vi "Washing_Machine.vi"() -> ()   [LabVIEW 2021]
uses:
  Controls/Queue_Operation_Select.ctl
  Controls/State_and_Data.ctl
  Controls/Timer_Operation_Select.ctl
  Controls/INI_Operation_Select.ctl
  <vilib>/Utility/file.llb/Read Delimited Spreadsheet (string).vi
  8107810c-38f5-4bb1-a673-e4c5686a5b40.vi
  Controls/Wash_Type.ctl
panel:
  out "Elapsed_Time":dbl=1044.1757565 caption="Elapsed Time"
  out "Wash_Complete?":bool caption="Wash Complete?"
  out "Dry_Water":bool
  out "Short_Wash/Soak":bool
  out "Cool_Down":bool
  out "Regular":bool
  out "Machine_Underweight":bool
  out "Machine_Overweight":bool
  out "Machine_Load":dbl(slide) caption="Machine Load" scale=0.0..15.0
  in  "Unload":bool
  in  "Stop_Wash":bool
  in  "Start_Wash":bool
  in  "Wash_Type":T1 caption="Wash Type" scale=0.0..2.0
  in  "Add_Clothes":bool
  in  "Clothes [Kg]":dbl min=0.0 max=15.0
  out "Error_Out":errorcluster
  in  "Error_In":errorcluster
  # "Load Status"
  # "Sequence"
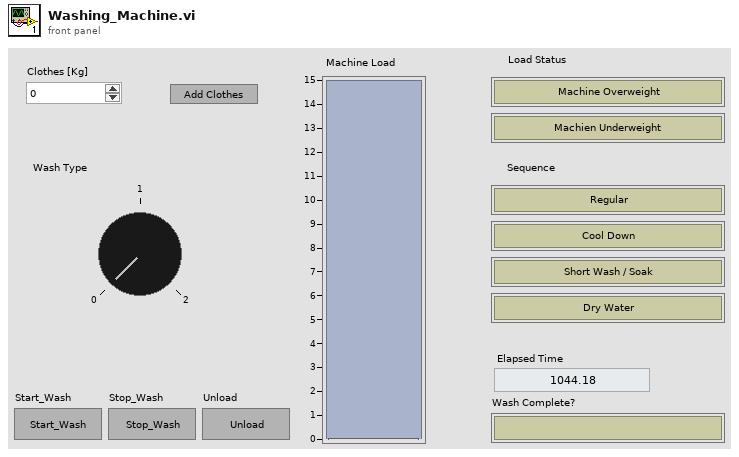
[diagram p1: front panel]
types:
  T1 = typedef "Wash_Type.ctl" = i32
  T2 = typedef "Timer_Operation_Select.ctl" = enum16{"Start_Timer", "Time_Out?", "Pause_Timer", "Stop_Timer"}
  T3 = typedef "State_and_Data.ctl" = cluster{"State":string, "Data":variant}
  T4 = typedef "Queue_Operation_Select.ctl" = enum16{"Obtain_Queue", "Enqueue", "Enqueue_First", "Enqueue_N", "Lossy_Enqueue", "Preview", "Queue_Status", "Dequeue", "Flush", "Release_Queue"}
  T5 = typedef "INI_Operation_Select.ctl" = enum16{"Initialize", "Read", "Write"}
  T6 = cluster{"Machine_Load":dbl, "Machine_Overweight":bool, "Machine_Underweight":bool, "Sequence":bool[], "Washing_Complete?":bool, "Disabled":enum8{"Enabled", "Disabled", "Disabled and Grayed Out"}, "Wash_Type":string, "Washing_Process":string[], "Process_Time":dbl[], "CSV_File_Path":path, "Current_Washing_Stage":i32, "Start?":bool, "Total_Washing_Stage":i32, "Washing_Process_F":bool[], "Machine_Load_Added":bool}
  T7 = enum8{"Enabled", "Disabled", "Disabled and Grayed Out"}
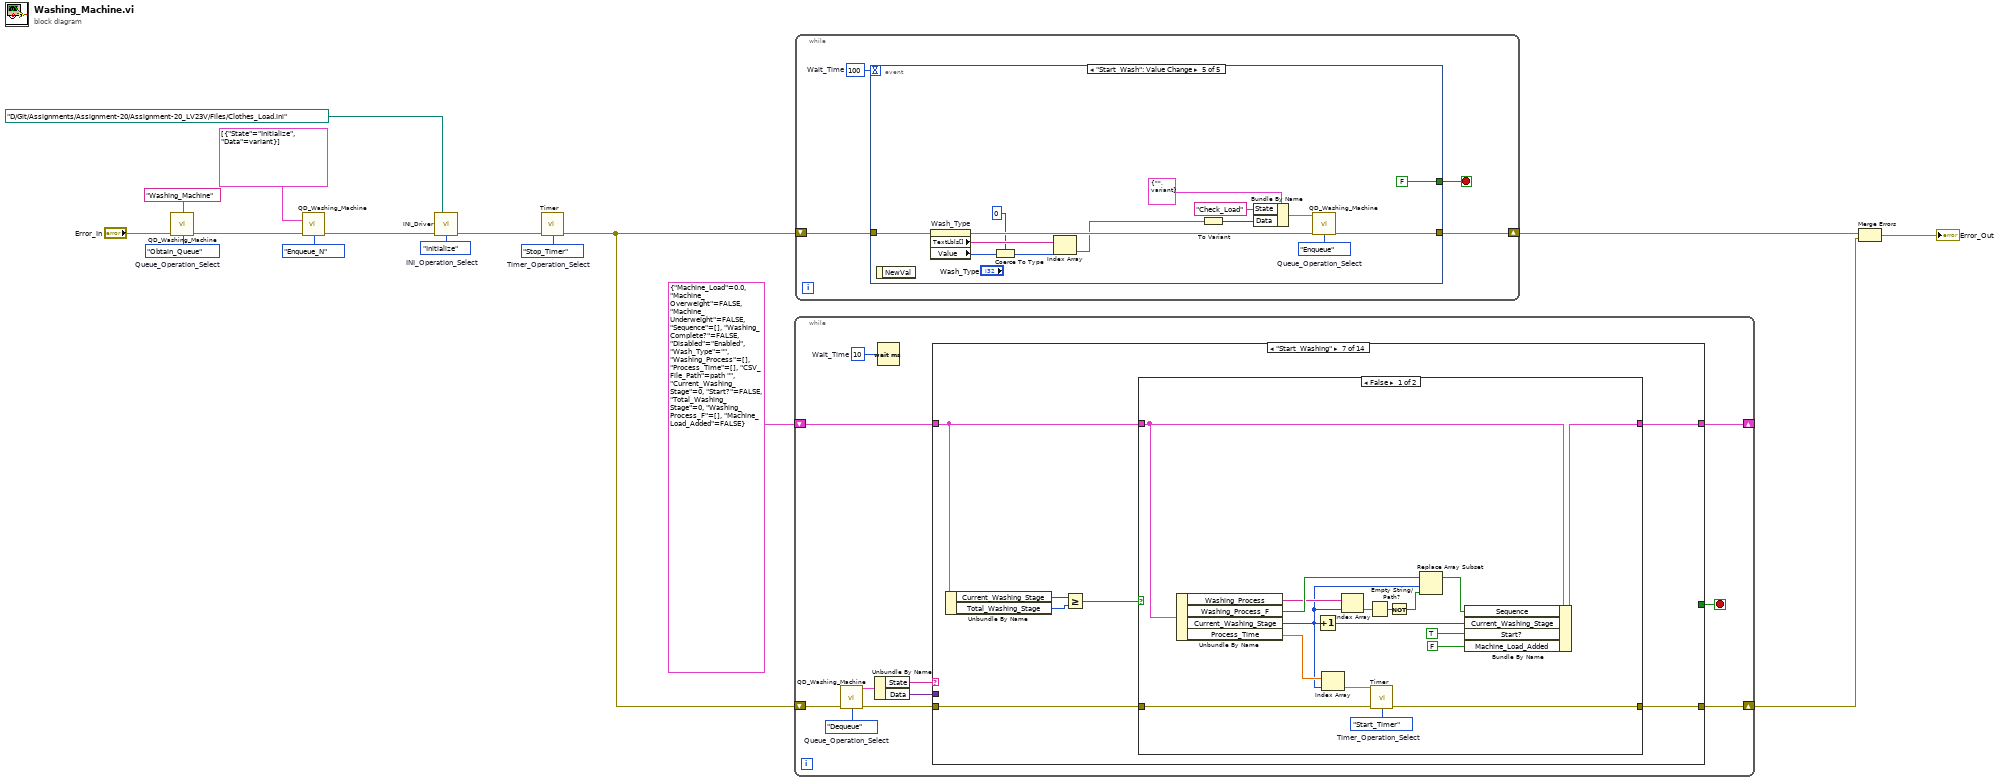
[diagram p0: block diagram]
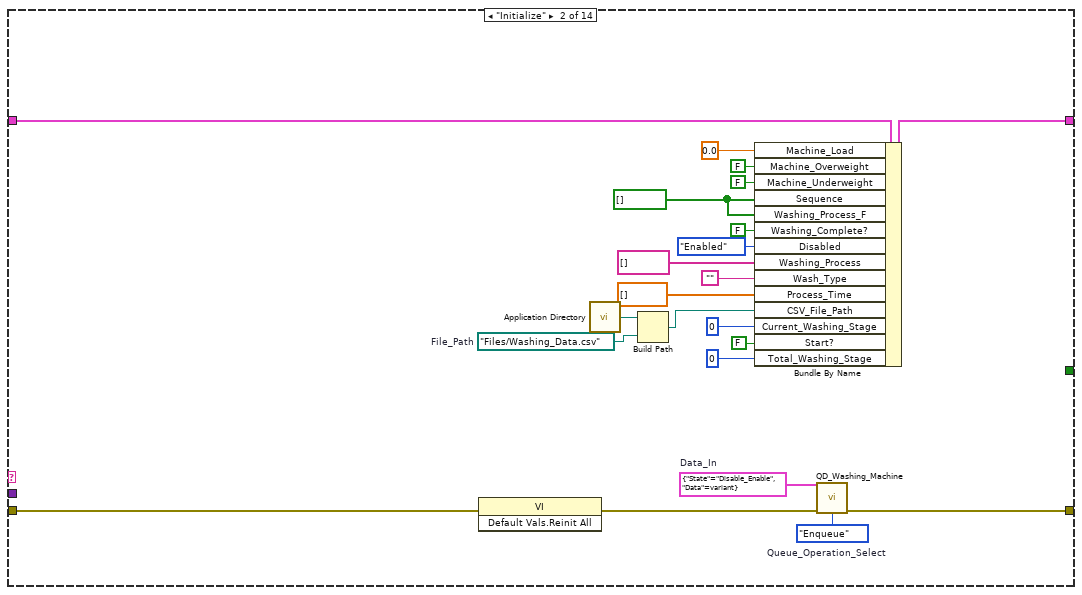
[diagram p3: hidden frame]
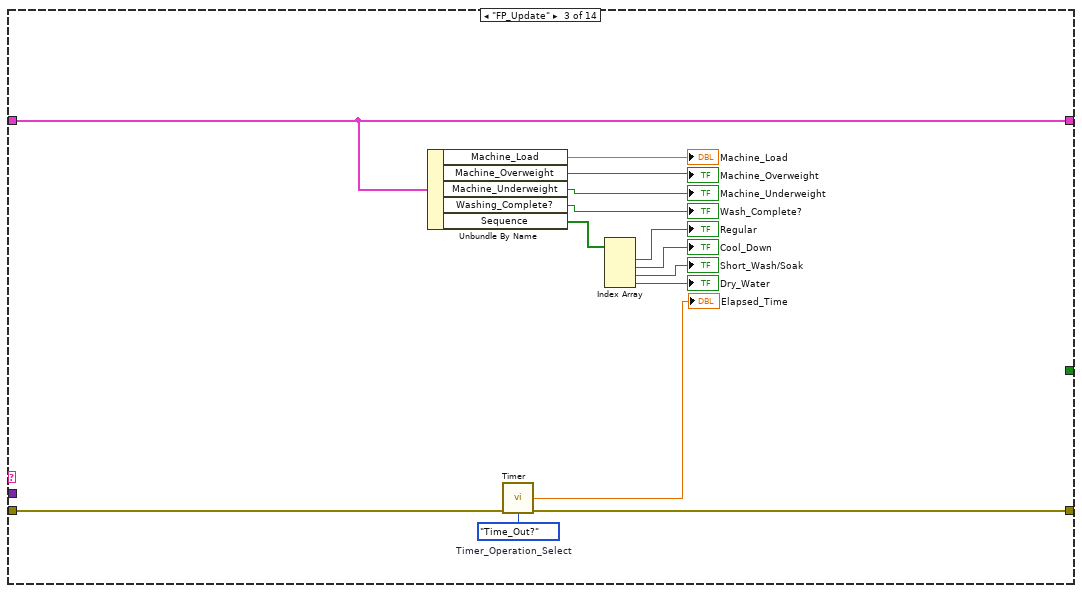
[diagram p4: hidden frame]
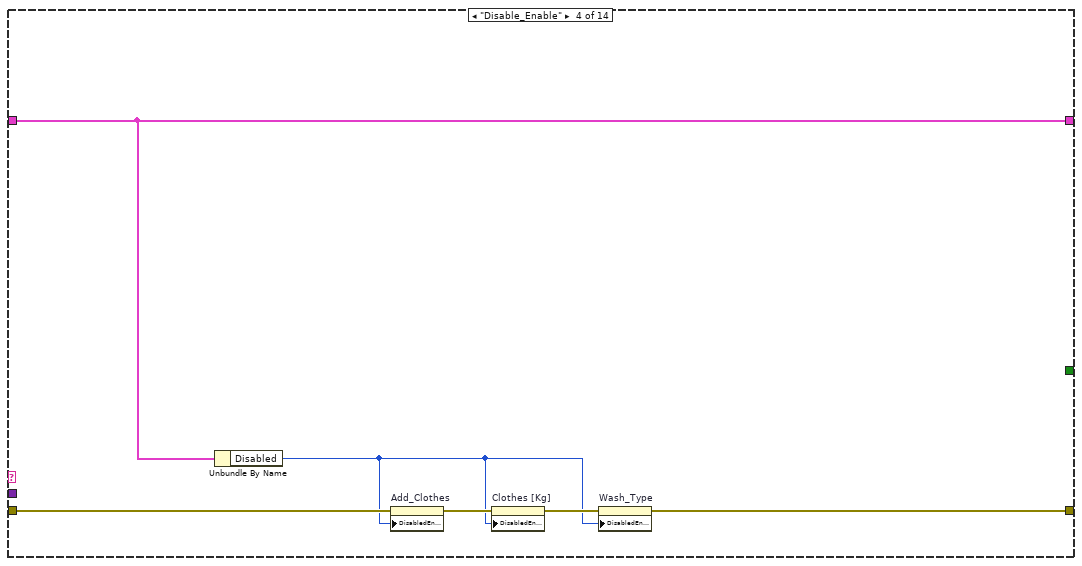
[diagram p5: hidden frame]
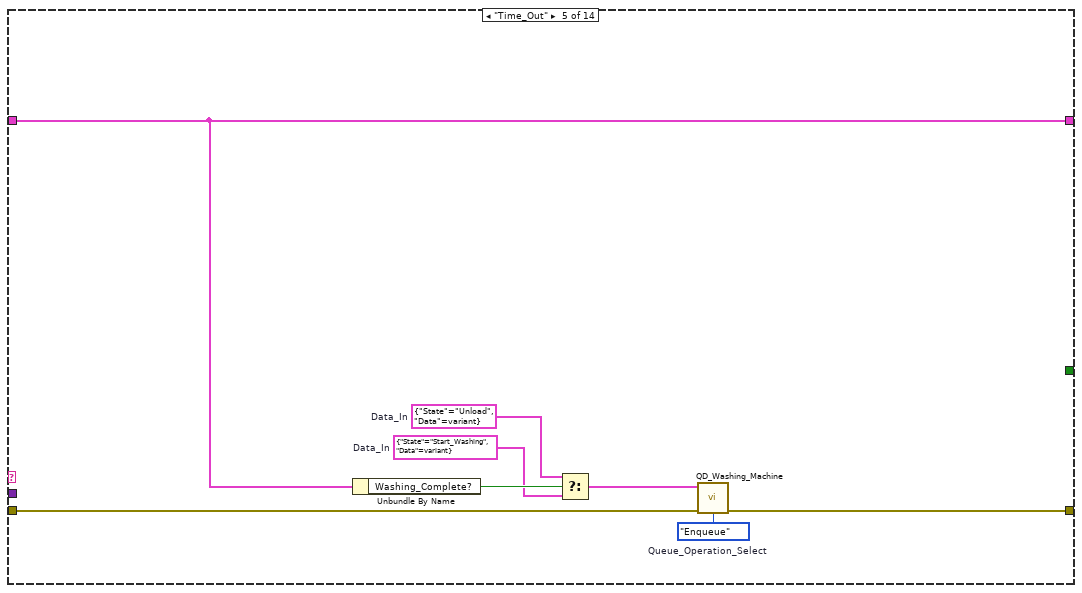
[diagram p6: hidden frame]
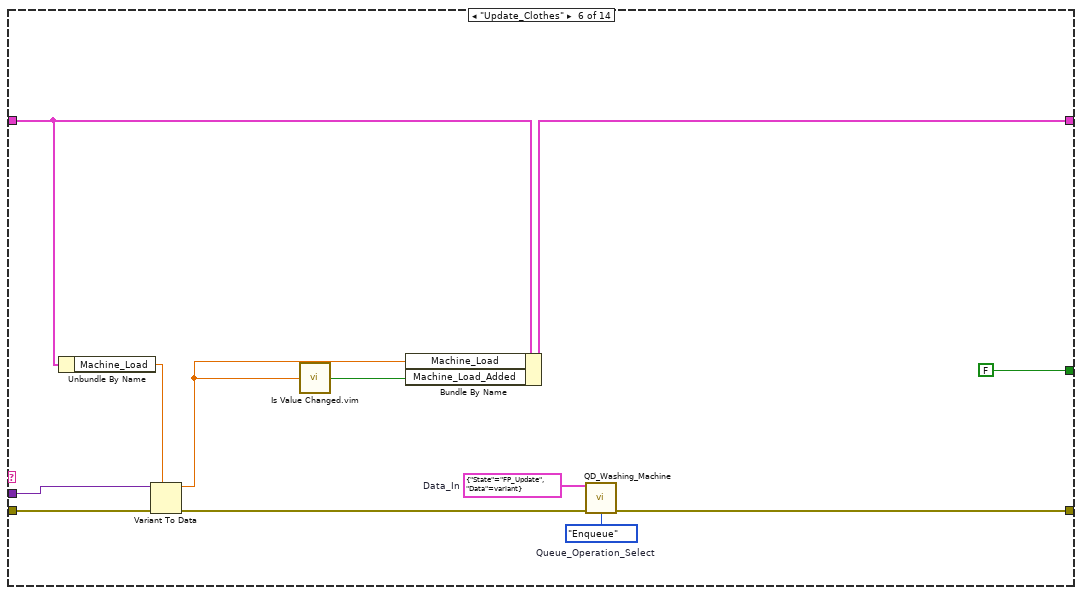
[diagram p7: hidden frame]
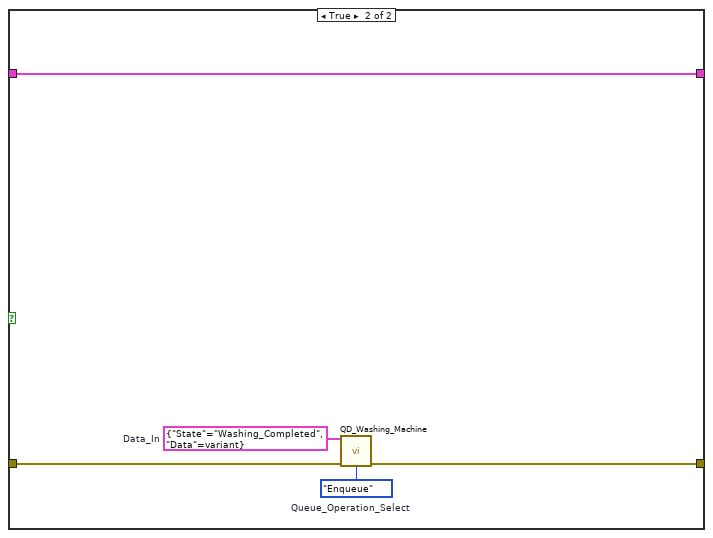
[diagram p8: hidden frame]
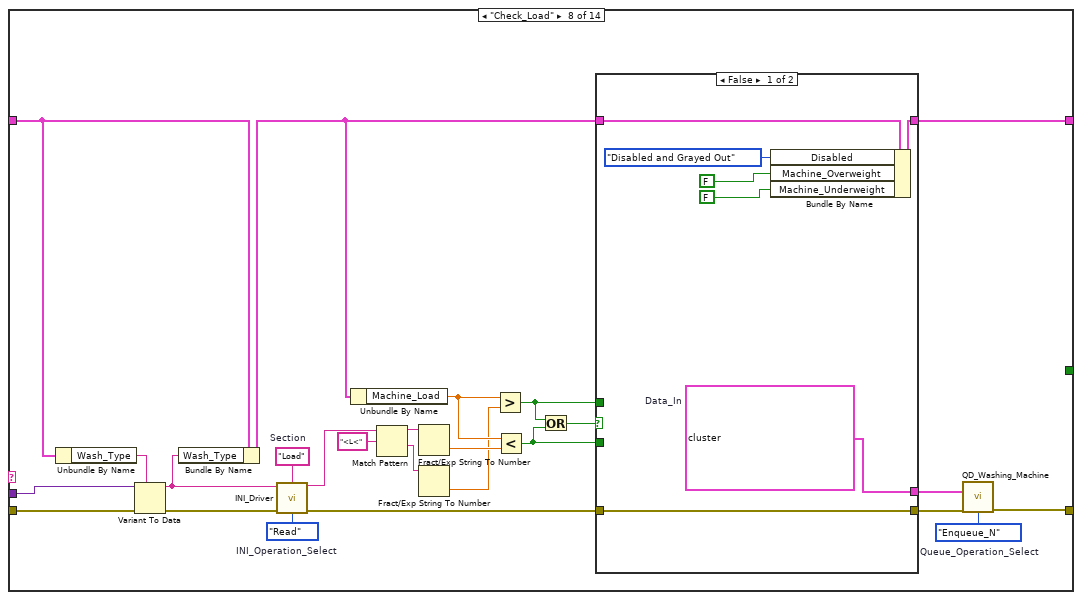
[diagram p9: hidden frame]
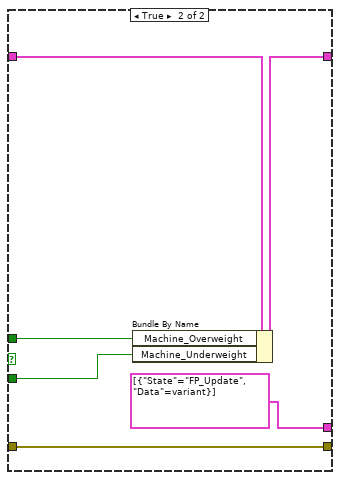
[diagram p10: hidden frame]
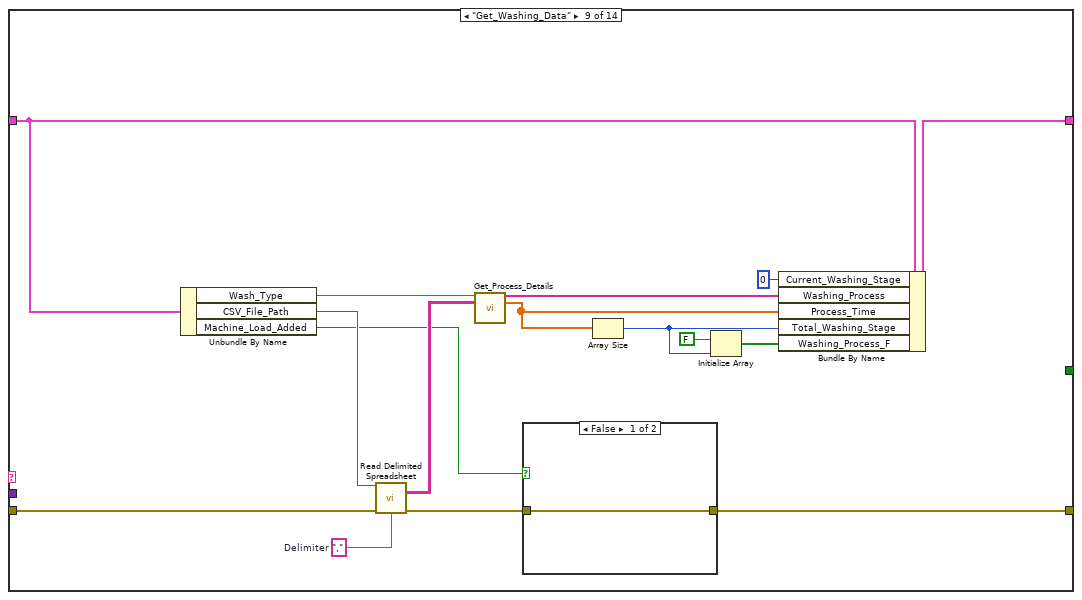
[diagram p11: hidden frame]
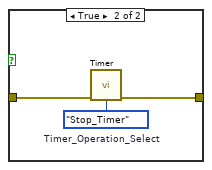
[diagram p12: hidden frame]
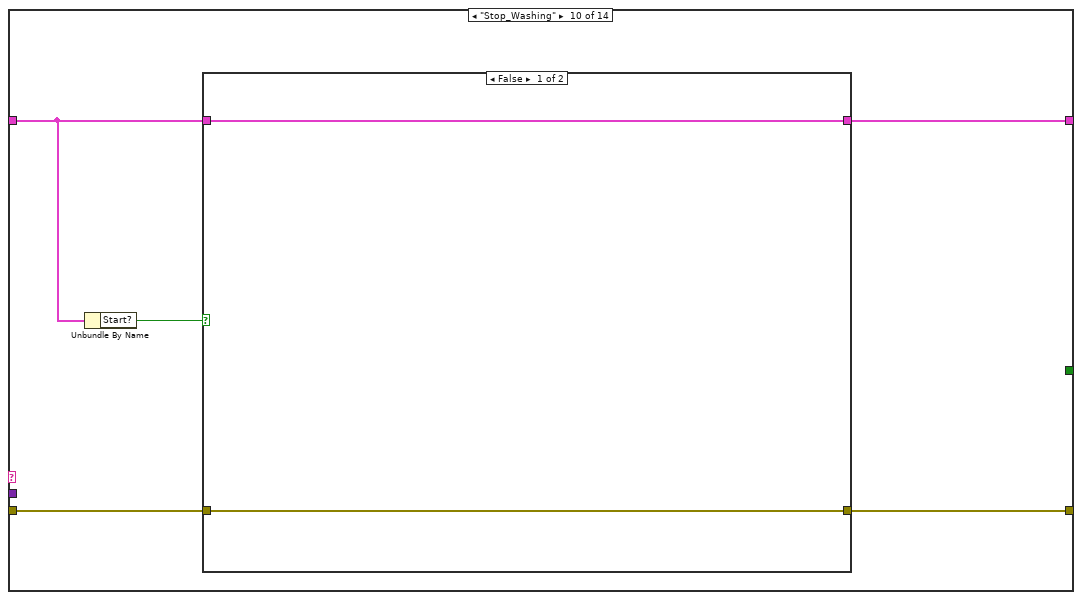
[diagram p13: hidden frame]
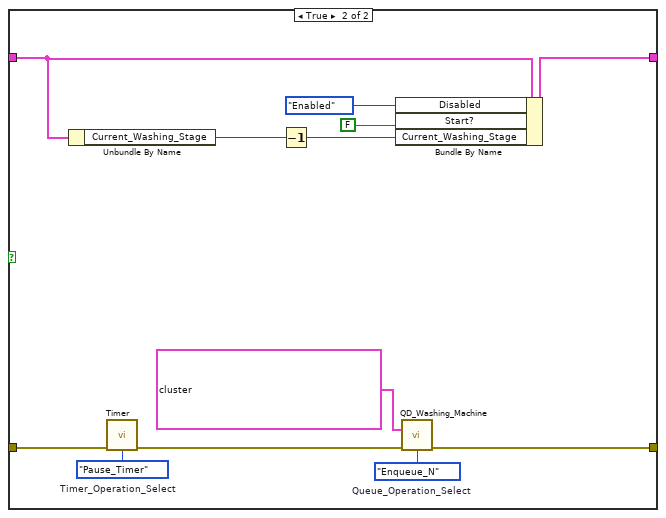
[diagram p14: hidden frame]
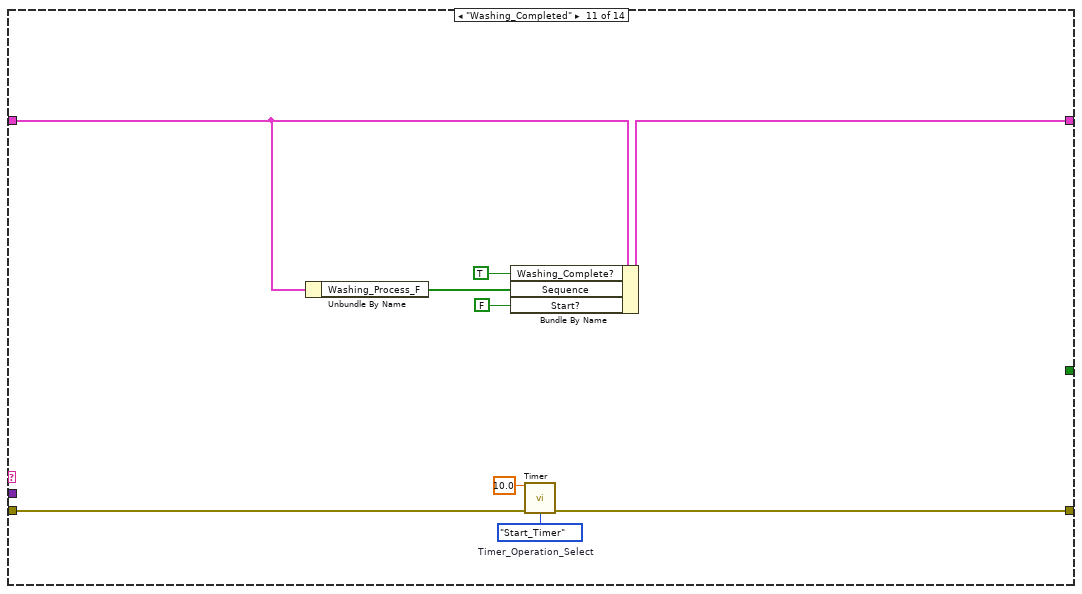
[diagram p15: hidden frame]
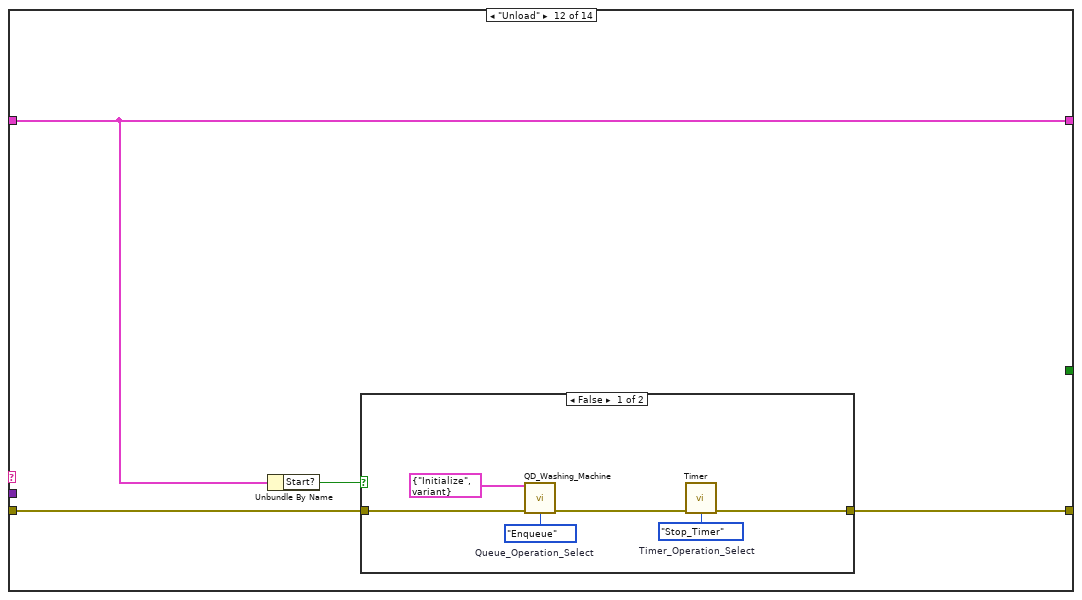
[diagram p16: hidden frame]
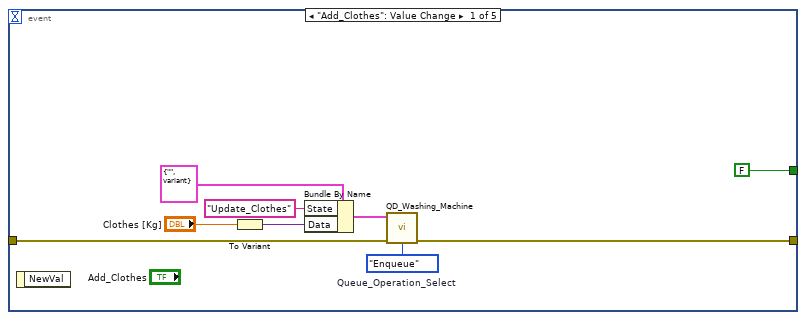
[diagram p20: hidden frame]
diagram:
  w3 = Timer_Operation_Select."Stop_Timer"  # Timer_Operation_Select
  w9 = INI_Operation_Select."Initialize"  # INI_Operation_Select
  w12 = Queue_Operation_Select."Obtain_Queue"  # Queue_Operation_Select
  n1 = call "QD_Washing_Machine.vi"("Queue_Name_In"="Washing_Machine", "Error_In"="Error_In", "Queue_Operation_Select"=w12) -> ("Error_Out"=w14:errorcluster)  [unwired: 10 in, 2 out]
  n2 = call "QD_Washing_Machine.vi"("Data_In"=T3[] [{"State"="Initialize", "Data"=variant}], "Error_In"=w14, "Queue_Operation_Select"=Queue_Operation_Select."Enqueue_N") -> ("Error_Out"=w7:errorcluster)  [unwired: 10 in, 2 out]
  n3 = call "INI_Driver.vi"("Config_File_Path"=path "D:/Git/Assignments/Assignment-20/Assignment-20_LV23V/Files/Clothes_Load.ini", "Error_Out"=w7, "INI_Operation_Select"=w9) -> ("Error_Out"=w10:errorcluster)  [unwired: 11 in, 1 out]
  n4 = call "Timer.vi"("Error_In"=w10, "Timer_Operation_Select"=w3) -> ("Error_Out"=w4:errorcluster)  [unwired: 10 in, 3 out]
  n5 = while {
    shift-right: [w26] -> w1
    shift-left: w4 -> [w27]
    shift-right: [w20] -> _
    shift-left: T6 {"Machine_Load"=0.0, "Machine_Overweight"=FALSE, "Machine_Underweight"=FALSE, "Sequence"=[], "Washing_Complete?"=FALSE, "Disabled"=enum."Enabled", "Wash_Type"="", "Washing_Process"=[], "Process_Time"=[], "CSV_File_Path"=path "", "Current_Washing_Stage"=0, "Start?"=FALSE, "Total_Washing_Stage"=0, "Washing_Process_F"=[], "Machine_Load_Added"=FALSE} -> [w19]
    stop <- w18 stop-if-true
    w17 = u32 10  # Wait_Time
    w24 = Queue_Operation_Select."Dequeue"  # Queue_Operation_Select
    n6 = call "QD_Washing_Machine.vi"("Error_In"=w27, "Queue_Operation_Select"=w24) -> ("Data_Out"=w23:T3, "Error_Out"=w25:errorcluster)  [unwired: 11 in, 1 out]
    n7 = Unbundle By Name(w23) -> ("State"=w22:string, "Data"=w21:variant)
    n8 = Wait (ms)(milliseconds to wait=w17) -> ()  [unwired: 1 out]
    n9 = case shown="\"Start_Washing\"" w22 {
      tunnel: w25 -> [w29 w51 w65 w71 w79 w91 w98 w145 w174 w183 w204 w210 w219 w221]
      tunnel: [w29 w33 w54 w69 w77 w85 w97 w130 w160 w181 w203 w209 w219 w221] -> w26
      tunnel: w21 -> [_ _ _ _ _ w88 _ w144 _ _ _ _ _ _]
      tunnel: [w28 w48 w64 w67 w78 w90 w96 w134 w170 w182 w206 w208 w218 w220] -> w20
      tunnel: w19 -> [w28 w50 w64 w67 w78 w87 w95 w143 w173 w180 w200 w208 w218 w220]
      tunnel: [_ _ _ _ _ FALSE _ _ _ _ _ _ _ _] -> w18
      frame "False", Default {
      }
      frame "Initialize" {
        w31 = T3 {"State"="Disable_Enable", "Data"=variant}  # Data_In
        w32 = Queue_Operation_Select."Enqueue"  # Queue_Operation_Select
        w37 = path "Files/Washing_Data.csv"  # File_Path
        w30 = bool[] [] ("Sequence")
        n10 = invoke class="VI" method="Default Vals.Reinit All"(error in=w51) -> (error out=w49:errorcluster)  [unwired: 2 in, 2 out]
        n11 = call <vilib>:"Application Directory.vi"() -> ("Application Directory"=w38:path)
        n12 = Build Path(base path=w38, name or relative path=w37) -> (appended path=w39:path)
        n13 = Bundle By Name(cluster=w50, "Machine_Load"=0.0, "Machine_Overweight"=FALSE, "Machine_Underweight"=FALSE, "Sequence"=w30, "Washing_Process_F"=w30, "Washing_Complete?"=FALSE, "Disabled"=T7."Enabled", "Washing_Process"=string[] [], "Wash_Type"="", "Process_Time"=dbl[] [], "CSV_File_Path"=w39, "Current_Washing_Stage"=0, "Start?"=FALSE, "Total_Washing_Stage"=0) -> (w48:T6)
        n14 = call "QD_Washing_Machine.vi"("Data_In"=w31, "Error_In"=w49, "Queue_Operation_Select"=w32) -> ("Error_Out"=w33:errorcluster)  [unwired: 10 in, 2 out]
      }
      frame "FP_Update" {
        w53 = Timer_Operation_Select."Time_Out?"  # Timer_Operation_Select
        n15 = Unbundle By Name(w64) -> ("Machine_Load"=→"Machine_Load":dbl, "Machine_Overweight"=→"Machine_Overweight":bool, "Machine_Underweight"=→"Machine_Underweight":bool, "Washing_Complete?"=→"Wash_Complete?":bool, "Sequence"=w59:bool[])
        n16 = call "Timer.vi"("Error_In"=w65, "Timer_Operation_Select"=w53) -> ("Time"=→"Elapsed_Time":dbl, "Error_Out"=w54:errorcluster)  [unwired: 10 in, 2 out]
        n17 = Index Array(array=w59) -> (element #1=→"Regular":bool, element #2=→"Cool_Down":bool, element #3=→"Short_Wash/Soak":bool, element #4=→"Dry_Water":bool)  [unwired: 4 in]
      }
      frame "Disable_Enable" {
        n18 = Unbundle By Name(w67) -> ("Disabled"=w66:T7)
        n19 = property on="Add_Clothes" class="Bool"(error in=w71, "DisabledEnum"=w66) -> (error out=w68:errorcluster)  [unwired: 1 in, 1 out]
        n20 = property on="Clothes [Kg]" class="DigNum (strict)"(error in=w68, "DisabledEnum"=w66) -> (error out=w70:errorcluster)  [unwired: 1 in, 1 out]
        n21 = property on="Wash_Type" class="Knob (strict)"(error in=w70, "DisabledEnum"=w66) -> (error out=w69:errorcluster)  [unwired: 1 in, 1 out]
      }
      frame "Time_Out" {
        w73 = T3 {"State"="Start_Washing", "Data"=variant}  # Data_In
        w74 = T3 {"State"="Unload", "Data"=variant}  # Data_In
        w76 = Queue_Operation_Select."Enqueue"  # Queue_Operation_Select
        n22 = Unbundle By Name(w78) -> ("Washing_Complete?"=w75:bool)
        n23 = Select(t=w74, s=w75, f=w73) -> (s? t:f=w72:T3)
        n24 = call "QD_Washing_Machine.vi"("Data_In"=w72, "Error_In"=w79, "Queue_Operation_Select"=w76) -> ("Error_Out"=w77:errorcluster)  [unwired: 10 in, 2 out]
      }
      frame "Update_Clothes" {
        w83 = T3 {"State"="FP_Update", "Data"=variant}  # Data_In
        w84 = Queue_Operation_Select."Enqueue"  # Queue_Operation_Select
        n25 = Unbundle By Name(w87) -> ("Machine_Load"=w86:dbl)
        n26 = Variant To Data(error in=w91, type=w86, Variant=w88) -> (data=w81:dbl, error out=w89:errorcluster)
        n27 = call "Is Value Changed.vim"("value"=w81) -> ("changed or first call?"=w80:bool)
        n28 = Bundle By Name(cluster=w87, "Machine_Load"=w81, "Machine_Load_Added"=w80) -> (w90:T6)
        n29 = call "QD_Washing_Machine.vi"("Data_In"=w83, "Error_In"=w89, "Queue_Operation_Select"=w84) -> ("Error_Out"=w85:errorcluster)  [unwired: 10 in, 2 out]
      }
      frame "Start_Washing" {
        n30 = Unbundle By Name(w95) -> ("Current_Washing_Stage"=w94:i32, "Total_Washing_Stage"=w93:i32)
        n31 = Greater Or Equal?(x=w94, y=w93) -> (x >= y?=w92:bool)
        n32 = case shown="False" w92 {
          tunnel: w98 -> [w115 w119]
          tunnel: w95 -> [w114 w120]
          tunnel: [w113 w118] -> w97
          tunnel: [w110 w120] -> w96
          frame False {
            w112 = Timer_Operation_Select."Start_Timer"  # Timer_Operation_Select
            n33 = Unbundle By Name(w114) -> ("Washing_Process"=w104:string[], "Washing_Process_F"=w109:bool[], "Current_Washing_Stage"=w103:i32, "Process_Time"=w108:dbl[])
            n34 = Increment(x=w103) -> (x+1=w105:i32)
            n35 = Index Array(array=w108, index=w103) -> (element=w111:dbl)
            n36 = Index Array(array=w104, index=w103) -> (element=w102:string)
            n37 = Empty String/Path?(string/path=w102) -> (empty?=w101:bool)
            n38 = call "Timer.vi"("Wait_Time"=w111, "Error_In"=w115, "Timer_Operation_Select"=w112) -> ("Error_Out"=w113:errorcluster)  [unwired: 9 in, 3 out]
            n39 = Not(x=w101) -> (.not. x?=w100:bool)
            n40 = Replace Array Subset(array=w109, new element=w100, index=w103) -> (w106:bool[])
            n41 = Bundle By Name(cluster=w114, "Sequence"=w106, "Current_Washing_Stage"=w105, "Start?"=TRUE, "Machine_Load_Added"=FALSE) -> (w110:T6)
          }
          frame True {
            w116 = Queue_Operation_Select."Enqueue"  # Queue_Operation_Select
            w117 = T3 {"State"="Washing_Completed", "Data"=variant}  # Data_In
            n42 = call "QD_Washing_Machine.vi"("Data_In"=w117, "Error_In"=w119, "Queue_Operation_Select"=w116) -> ("Error_Out"=w118:errorcluster)  [unwired: 10 in, 2 out]
          }
        }
      }
      frame "Check_Load" {
        w132 = Queue_Operation_Select."Enqueue_N"  # Queue_Operation_Select
        w140 = "Load"  # Section
        w141 = INI_Operation_Select."Read"  # INI_Operation_Select
        n43 = Unbundle By Name(w143) -> ("Wash_Type"=w142:string)
        n44 = Variant To Data(error in=w145, type=w142, Variant=w144) -> (data=w128:string, error out=w129:errorcluster)
        n45 = Bundle By Name(cluster=w143, "Wash_Type"=w128) -> (w133:T6)
        n46 = call "INI_Driver.vi"("Key"=w128, "Section"=w140, "Error_Out"=w129, "INI_Operation_Select"=w141) -> ("Data_Out"=w139:string, "Error_Out"=w135:errorcluster)  [unwired: 10 in]
        n47 = Unbundle By Name(w133) -> ("Machine_Load"=w127:dbl)
        n48 = Match Pattern(string=w139, regular expression="<L<") -> (before substring=w137:string, after substring=w136:string)  [unwired: 1 in, 2 out]
        n49 = Fract/Exp String To Number(string=w137) -> (number=w126:dbl)  [unwired: 3 in, 1 out]
        n50 = Fract/Exp String To Number(string=w136) -> (number=w125:dbl)  [unwired: 3 in, 1 out]
        n51 = Greater?(x=w127, y=w125) -> (0:w123:bool)
        n52 = Less?(x=w127, y=w126) -> (x < y?=w122:bool)
        n53 = Or(x=w123, y=w122) -> (x .or. y?=w124:bool)
        n54 = case shown="False" w124 {
          tunnel: [w151 w158] -> w131
          tunnel: w135 -> [w151 w158]
          tunnel: [w150 w156] -> w134
          tunnel: w133 -> [w152 w157]
          tunnel: w123 -> [_ w155]
          tunnel: w122 -> [_ w154]
          tunnel: [w148 T3[] [{"State"="FP_Update", "Data"=variant}] ("Data_In")] -> w121
          frame False {
            w148 = T3[] [{"State"="Disable_Enable", "Data"=variant}, {"State"="Get_Washing_Data", "Data"=variant}, {"State"="Start_Washing", "Data"=variant}]  # Data_In
            n55 = Bundle By Name(cluster=w152, "Disabled"=T7."Disabled and Grayed Out", "Machine_Overweight"=FALSE, "Machine_Underweight"=FALSE) -> (w150:T6)
          }
          frame True {
            n56 = Bundle By Name(cluster=w157, "Machine_Overweight"=w155, "Machine_Underweight"=w154) -> (w156:T6)
          }
        }
        n57 = call "QD_Washing_Machine.vi"("Data_In"=w121, "Error_In"=w131, "Queue_Operation_Select"=w132) -> ("Error_Out"=w130:errorcluster)  [unwired: 10 in, 2 out]
      }
      frame "Get_Washing_Data" {
        w168 = ","  # Delimiter
        n58 = Unbundle By Name(w173) -> ("Wash_Type"=w172:string, "CSV_File_Path"=w169:path, "Machine_Load_Added"=w159:bool)
        n59 = call-poly <vilib>:"Read Delimited Spreadsheet.vi"("file path (dialog if empty)"=w169, "error in (no error)"=w174, "delimiter (\\t)"=w168) -> ("all rows"=w171:string[][], "error out"=w167:errorcluster)  [unwired: 7 in, 4 out]
        n60 = call "Get_Process_Details.vi"("Wash_Type"=w172, "Process_Data"=w171) -> ("Process"=w165:string[], "Time"=w166:dbl[])  [unwired: 12 in]
        n61 = case shown="False" w159 {
          tunnel: w167 -> [w175 w178]
          tunnel: [w175 w177] -> w160
          frame False {
          }
          frame True {
            w176 = Timer_Operation_Select."Stop_Timer"  # Timer_Operation_Select
            n62 = call "Timer.vi"("Error_In"=w178, "Timer_Operation_Select"=w176) -> ("Error_Out"=w177:errorcluster)  [unwired: 10 in, 3 out]
          }
        }
        n63 = Array Size(array=w166) -> (size(s)=w163:i32)
        n64 = Initialize Array(FALSE ("Sequence"), w163) -> (w164:bool[])
        n65 = Bundle By Name(cluster=w173, "Current_Washing_Stage"=0, "Washing_Process"=w165, "Process_Time"=w166, "Total_Washing_Stage"=w163, "Washing_Process_F"=w164) -> (w170:T6)
      }
      frame "Stop_Washing" {
        n66 = Unbundle By Name(w180) -> ("Start?"=w179:bool)
        n67 = case shown="False" w179 {
          tunnel: w183 -> [w184 w197]
          tunnel: [w185 w196] -> w182
          tunnel: [w184 w192] -> w181
          tunnel: w180 -> [w185 w188]
          frame False {
          }
          frame True {
            w191 = Queue_Operation_Select."Enqueue_N"  # Queue_Operation_Select
            w193 = Timer_Operation_Select."Pause_Timer"  # Timer_Operation_Select
            n68 = Unbundle By Name(w188) -> ("Current_Washing_Stage"=w187:i32)
            n69 = call "Timer.vi"("Error_In"=w197, "Timer_Operation_Select"=w193) -> ("Error_Out"=w194:errorcluster)  [unwired: 10 in, 3 out]
            n70 = Decrement(x=w187) -> (x-1=w186:i32)
            n71 = Bundle By Name(cluster=w188, "Disabled"=T7."Enabled", "Start?"=FALSE, "Current_Washing_Stage"=w186) -> (w196:T6)
            n72 = call "QD_Washing_Machine.vi"("Data_In"=T3[] [{"State"="Disable_Enable", "Data"=variant}, {"State"="FP_Update", "Data"=variant}], "Error_In"=w194, "Queue_Operation_Select"=w191) -> ("Error_Out"=w192:errorcluster)  [unwired: 10 in, 2 out]
          }
        }
      }
      frame "Washing_Completed" {
        w202 = Timer_Operation_Select."Start_Timer"  # Timer_Operation_Select
        n73 = Unbundle By Name(w200) -> ("Washing_Process_F"=w199:bool[])
        n74 = Bundle By Name(cluster=w200, "Washing_Complete?"=TRUE, "Sequence"=w199, "Start?"=FALSE) -> (w206:T6)
        n75 = call "Timer.vi"("Wait_Time"=10.0, "Error_In"=w204, "Timer_Operation_Select"=w202) -> ("Error_Out"=w203:errorcluster)  [unwired: 9 in, 3 out]
      }
      frame "Unload" {
        n76 = Unbundle By Name(w208) -> ("Start?"=w207:bool)
        n77 = case shown="False" w207 {
          tunnel: w210 -> [w216 w217]
          tunnel: [w212 w217] -> w209
          frame False {
            w211 = Timer_Operation_Select."Stop_Timer"  # Timer_Operation_Select
            w214 = Queue_Operation_Select."Enqueue"  # Queue_Operation_Select
            n78 = call "QD_Washing_Machine.vi"("Data_In"=T3 {"State"="Initialize", "Data"=variant}, "Error_In"=w216, "Queue_Operation_Select"=w214) -> ("Error_Out"=w215:errorcluster)  [unwired: 10 in, 2 out]
            n79 = call "Timer.vi"("Error_In"=w215, "Timer_Operation_Select"=w211) -> ("Error_Out"=w212:errorcluster)  [unwired: 10 in, 3 out]
          }
          frame True {
          }
        }
      }
      frame "Error" {
      }
      frame "Exit" {
      }
    }
  }
  n80 = while {
    shift-right: [w225] -> w15
    shift-left: w4 -> [w224]
    stop <- w223 stop-if-true
    w222 = 100  # Wait_Time
    n81 = event shown="[4] \"Start_Wash\": Value Change" {
      selector: _ -> [_ _ _ _ _]
      dyn-events: _ -> [_ _ _ _ _]
      timeout: w222 -> [_ _ _ _ _]
      tunnel: [w233 w241 w254 w261 w275] -> w225
      tunnel: w224 -> [w234 w242 w255 w262 w276]
      tunnel: [FALSE _ FALSE FALSE FALSE] -> w223
      event "Add_Clothes": Value Change {
        w232 = Queue_Operation_Select."Enqueue"  # Queue_Operation_Select
        n82 = event-data() -> ()  [unwired: 1 in, 1 out]
        n83 = To Variant(anything="Clothes [Kg]") -> (Variant=w227:variant)
        n84 = Bundle By Name(cluster=T3 {"State"="", "Data"=variant} ("State_and_Data"), "State"="Update_Clothes", "Data"=w227) -> (w229:T3)
        n85 = call "QD_Washing_Machine.vi"("Data_In"=w229, "Error_In"=w234, "Queue_Operation_Select"=w232) -> ("Error_Out"=w233:errorcluster)  [unwired: 10 in, 2 out]
      }
      event Timeout {
        w239 = Timer_Operation_Select."Time_Out?"  # Timer_Operation_Select
        w240 = Queue_Operation_Select."Enqueue"  # Queue_Operation_Select
        n86 = event-data() -> ()  [unwired: 1 in, 2 out]
        n87 = call "Timer.vi"("Error_In"=w242, "Timer_Operation_Select"=w239) -> ("Time_Out?"=w237:bool, "Error_Out"=w235:errorcluster)  [unwired: 10 in, 2 out]
        n88 = case shown="True" w237 {
          tunnel: [T3 {"State"="FP_Update", "Data"=variant} ("f") T3 {"State"="Time_Out", "Data"=variant} ("Data_In")] -> w238
          tunnel: [w244 w246] -> w236
          tunnel: w235 -> [w244 w247]
          frame False {
          }
          frame True {
            w245 = Timer_Operation_Select."Stop_Timer"  # Timer_Operation_Select
            n89 = call "Timer.vi"("Error_In"=w247, "Timer_Operation_Select"=w245) -> ("Error_Out"=w246:errorcluster)  [unwired: 10 in, 3 out]
          }
        }
        n90 = call "QD_Washing_Machine.vi"("Data_In"=w238, "Error_In"=w236, "Queue_Operation_Select"=w240) -> ("Error_Out"=w241:errorcluster)  [unwired: 10 in, 2 out]
      }
      event "Stop_Wash": Value Change {
        w253 = Queue_Operation_Select."Enqueue"  # Queue_Operation_Select
        n91 = event-data() -> ()  [unwired: 1 in, 1 out]
        n92 = Bundle By Name(cluster=T3 {"State"="", "Data"=variant} ("State_and_Data"), "State"="Stop_Washing") -> (w251:T3)
        n93 = call "QD_Washing_Machine.vi"("Data_In"=w251, "Error_In"=w255, "Queue_Operation_Select"=w253) -> ("Error_Out"=w254:errorcluster)  [unwired: 10 in, 2 out]
      }
      event "Unload": Value Change {
        w260 = Queue_Operation_Select."Enqueue"  # Queue_Operation_Select
        n94 = event-data() -> ()  [unwired: 1 in, 1 out]
        n95 = Bundle By Name(cluster=T3 {"State"="", "Data"=variant} ("State_and_Data"), "State"="Unload") -> (w258:T3)
        n96 = call "QD_Washing_Machine.vi"("Data_In"=w258, "Error_In"=w262, "Queue_Operation_Select"=w260) -> ("Error_Out"=w261:errorcluster)  [unwired: 10 in, 2 out]
      }
      event "Start_Wash": Value Change {
        w274 = Queue_Operation_Select."Enqueue"  # Queue_Operation_Select
        n97 = event-data() -> ()  [unwired: 1 in, 1 out]
        n98 = property on="Wash_Type" class="Knob (strict)"(error in=w276) -> (error out=w268:errorcluster, "TextLbls[]"=w267:string[], "Value"=w265:T1)  [unwired: 1 in, 1 out]
        n99 = Coerce To Type(0:w265, 1:0) -> (2:w264:i32)
        n100 = Index Array(array=w267, index=w264) -> (element=w266:string)
        n101 = To Variant(anything=w266) -> (Variant=w270:variant)
        n102 = Bundle By Name(cluster=T3 {"State"="", "Data"=variant} ("State_and_Data"), "State"="Check_Load", "Data"=w270) -> (w272:T3)
        n103 = call "QD_Washing_Machine.vi"("Data_In"=w272, "Error_In"=w268, "Queue_Operation_Select"=w274) -> ("Error_Out"=w275:errorcluster)  [unwired: 10 in, 2 out]
      }
    }
  }
  n104 = Merge Errors(w15, w1) -> (→"Error_Out":errorcluster)
